vi "E443X_ESG_VSG_OPC.vi"(8 "error in (no error)":errorcluster, 9 "Maximum Time (10000ms)":u32=10000, 10 "Wait (1000ms)":u32=1000, 11 "VISA resource name":refnum<visa-resource-name>) -> (0 "error out":errorcluster, 3 "VISA resource name out":refnum<visa-resource-name>)   [LabVIEW 2015]
doc: "Waits for the current operation to finish. This VI should be called after Initiate VI.\n\n<B>Note:</B> \n\nUse this VI only with other low-level VIs. The high-level VIs automatically incorporate this functionality. This VI does not check the instrument status."
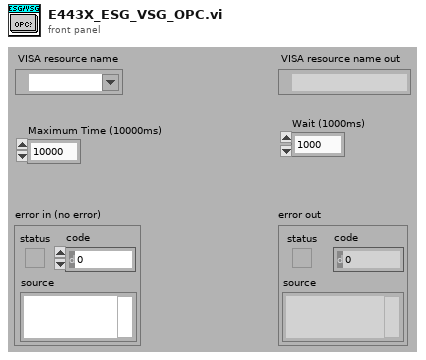
[diagram p1: front panel]
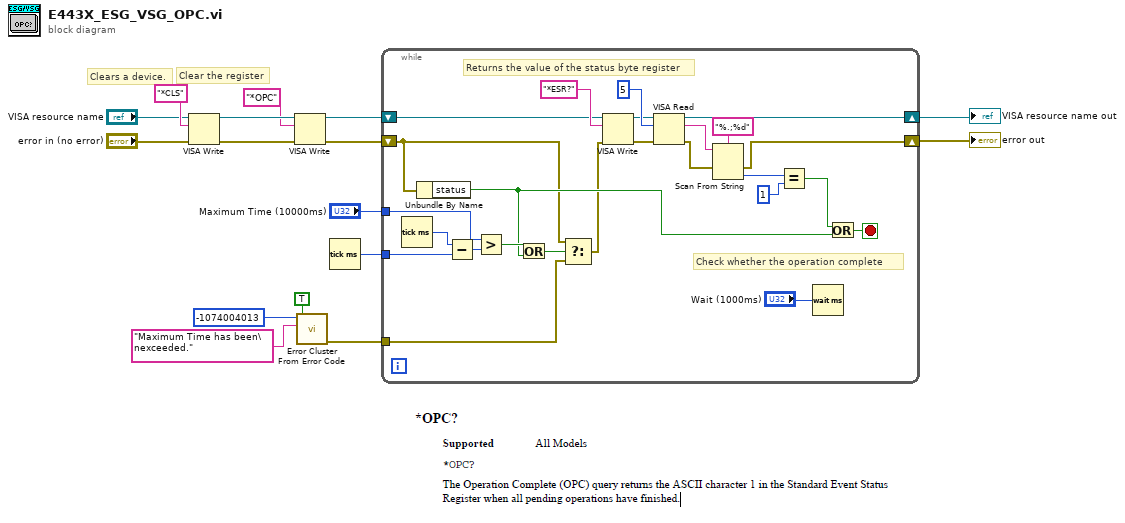
[diagram p0: block diagram]
diagram:
  # "Clears a device."
  # "Clear the register"
  n1 = VISA Write(VISA resource name="VISA resource name", write buffer="*CLS", error in (no error)="error in (no error)") -> (VISA resource name out=w6:refnum<visa-resource-name>, error out=w7:errorcluster)  [unwired: 1 out]
  n2 = VISA Write(VISA resource name=w6, write buffer="*OPC", error in (no error)=w7) -> (VISA resource name out=w5:refnum<visa-resource-name>, error out=w4:errorcluster)  [unwired: 1 out]
  n3 = call <vilib>:"Error Cluster From Error Code.vi"("show call chain? (False)"=TRUE, "error message (\"\")"="Maximum Time has been\nexceeded." ("error message (\"\")"), "error code (0)"=-1074004013) -> ("error out"=w10:errorcluster)  [unwired: 6 in]
  n4 = Tick Count (ms)() -> (millisecond timer value=w15:u32)
  n5 = while {
    tunnel: "Maximum Time (10000ms)" -> [w28]
    tunnel: w15 -> [w32]
    tunnel: w10 -> [w23]
    shift-right: [w30] -> w8
    shift-left: w4 -> [w21]
    shift-right: [w39] -> w9
    shift-left: w5 -> [w36]
    stop <- w29 stop-if-true
    # "Check whether the operation complete"
    # "Returns the value of the status byte register"
    n6 = Tick Count (ms)() -> (millisecond timer value=w33:u32)
    n7 = Unbundle By Name(w21) -> ("status"=w24:bool)
    n8 = Subtract(x=w33, y=w32) -> (x-y=w27:u32)
    n9 = Greater?(x=w28, y=w27) -> (0:w26:bool)
    n10 = Or(x=w26, y=w24) -> (x .or. y?=w25:bool)
    n11 = Select(t=w21, s=w25, f=w23) -> (s? t:f=w22:errorcluster)
    n12 = VISA Write(VISA resource name=w36, write buffer="*ESR?", error in (no error)=w22) -> (VISA resource name out=w34:refnum<visa-resource-name>, error out=w35:errorcluster)  [unwired: 1 out]
    n13 = VISA Read(VISA resource name=w34, byte count=u32 5, error in (no error)=w35) -> (VISA resource name out=w39:refnum<visa-resource-name>, read buffer=w41:string, error out=w31:errorcluster)  [unwired: 1 out]
    n14 = Scan From String(format string="%.;%d", input string=w41, error in=w31) -> (error out=w30:errorcluster, output 1=w19:i32)  [unwired: 2 in, 2 out]
    n15 = Equal?(x=w19, y=1 ("index")) -> (x = y?=w17:bool)
    n16 = Wait (ms)(milliseconds to wait="Wait (1000ms)") -> ()  [unwired: 1 out]
    n17 = Or(x=w17, y=w24) -> (x .or. y?=w29:bool)
  }
  "error out" <- w8
  "VISA resource name out" <- w9
